vi "Print Report.vi"(0 "report in":refnum<class "NI_Standard Report.lvclass">, 5 "printer name (default)":string, 9 "number of copies (1)":i32=1, 11 "error in (no error)":errorcluster) -> (4 "report out":refnum<class "NI_Standard Report.lvclass">, 15 "error out":errorcluster)   [LabVIEW 2015, in "NI_Standard Report.lvclass"]
doc: "Prints a report to a designated printer or to the default printer on the computer."
uses:
  <vilib>/Utility/NIReport.llb/Standard Report/NI_Standard Report.lvclass
  <vilib>/Utility/NIReport.llb/Standard Report/NI_Standard Report.lvclass/NI_Standard Report.ctl
  <vilib>/Utility/NIReport.llb/NI_ReportGenerationCore.lvlib
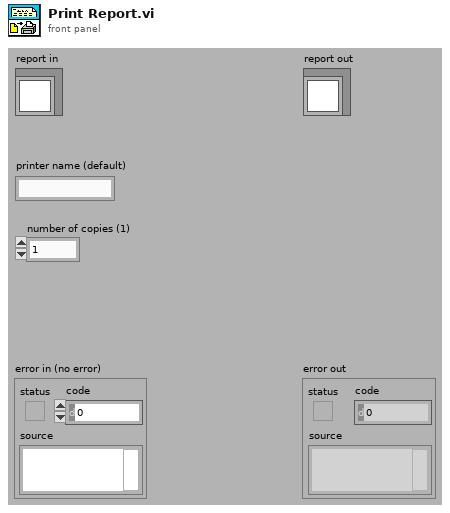
[diagram p1: front panel]
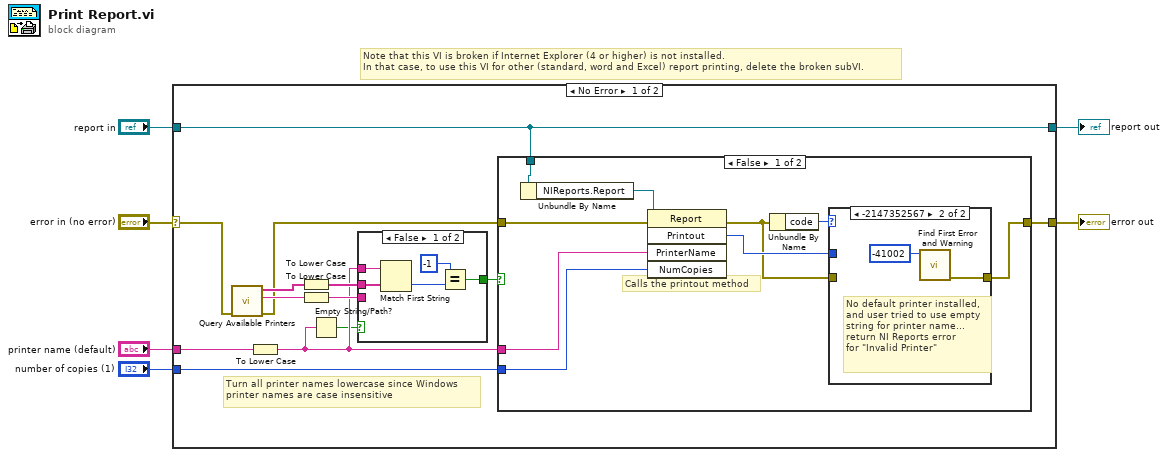
[diagram p0: block diagram]
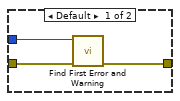
[diagram p2: hidden frame]
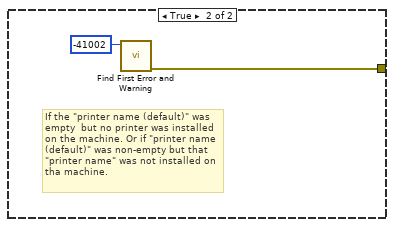
[diagram p3: hidden frame]
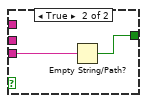
[diagram p4: hidden frame]
diagram:
  # "Note that this VI is broken if Internet Explorer (4 or higher) is not installed.\nIn that case, to use this VI for other (standard, word and Excel) report printing, delete the broken subVI."
  n1 = case shown="No Error" "error in (no error)" {
    selector: "error in (no error)" -> [w7 w44]
    tunnel: [w8 w44] -> w5
    tunnel: [w9 w43] -> w3
    tunnel: "report in" -> [w9 w43]
    tunnel: "printer name (default)" -> [w11 _]
    tunnel: "number of copies (1)" -> [w10 _]
    frame No Error {
      # "Turn all printer names lowercase since Windows\nprinter names are case insensitive"
      n2 = call <vilib>:"Query Available Printers.vi"("error in (no error)"=w7) -> ("error out"=w14:errorcluster, "default printer"=w16:string, "system configured printers"=w15:string[])  [unwired: 8 out]
      n3 = To Lower Case(string=w11) -> (all lower case string=w17:string)
      n4 = To Lower Case(string=w15) -> (all lower case string=w18:string[])
      n5 = To Lower Case(string=w16) -> (all lower case string=w19:string)
      n6 = Empty String/Path?(string/path=w17) -> (empty?=w12:bool)
      n7 = case shown="False" w12 {
        tunnel: w17 -> [w36 _]
        tunnel: [w37 w42] -> w13
        tunnel: w18 -> [w38 _]
        tunnel: w19 -> [_ w41]
        frame False {
          n8 = Match First String(2:w38, 3:w36) -> (0:w40:i32)  [unwired: 1 out]
          n9 = Equal?(x=-1 ("y"), y=w40) -> (x = y?=w37:bool)
        }
        frame True {
          n10 = Empty String/Path?(string/path=w41) -> (empty?=w42:bool)
        }
      }
      n11 = case shown="False" w13 {
        tunnel: w10 -> [w28 _]
        tunnel: [w27 w35] -> w8
        tunnel: w14 -> [w23 _]
        tunnel: w17 -> [w26 _]
        tunnel: w9 -> [w22 _]
        frame False {
          # "Calls the printout method"
          n12 = Unbundle By Name(w22) -> ("NIReports.Report"=w20:refnum<k7>)
          n13 = invoke class="Report" method="Printout"(reference=w20, error in=w23, "PrinterName"=w26, "NumCopies"=w28) -> (error out=w21:errorcluster, "Printout"=w24:i32)  [unwired: 1 in, 3 out]
          n14 = Unbundle By Name(w21) -> ("code"=w25:i32)
          n15 = case shown="-2147352567" w25 {
            tunnel: w21 -> [w31 _]
            tunnel: w24 -> [w30 _]
            tunnel: [w29 w33] -> w27
            frame Default {
              n16 = call <vilib>:"Find First Error and Warning.vi"("error in (no error)"=w31, "error code"=w30) -> ("error out"=w29:errorcluster)  [unwired: 1 in, 4 out]
            }
            frame -2147352567 {
              # "No default printer installed,\nand user tried to use empty\nstring for printer name...\nreturn NI Reports error\nfor \"Invalid Printer\""
              n17 = call <vilib>:"Find First Error and Warning.vi"("error code"=-41002) -> ("error out"=w33:errorcluster)  [unwired: 2 in, 4 out]
            }
          }
        }
        frame True {
          # "If the \"printer name (default)\" was empty  but no printer was installed on the machine. Or if \"printer name (default)\" was non-empty but that \"printer name\" was not installed on tha machine."
          n18 = call <vilib>:"Find First Error and Warning.vi"("error code"=-41002) -> ("error out"=w35:errorcluster)  [unwired: 1 in, 5 out]
        }
      }
    }
    frame Error {
    }
  }
  "error out" <- w5
  "report out" <- w3
